vi "Traverse_Space_channels.vi"() -> (0 "Channel Names":string[](array[string]))   [LabVIEW 2010]
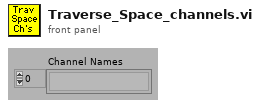
[diagram p1: front panel]
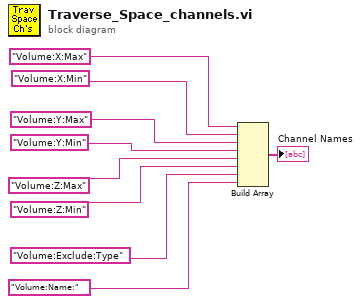
[diagram p0: block diagram]
diagram:
  n1 = Build Array("Volume:X:Max", "Volume:X:Min", "Volume:Y:Max", "Volume:Y:Min", "Volume:Z:Max", "Volume:Z:Min", "Volume:Exclude:Type", "Volume:Name:") -> (→"Channel Names":string[])
